vi "publisher.vi"() -> ()   [LabVIEW 2022 SP3]
uses:
  Global 1.vi
panel:
  in  "String":string
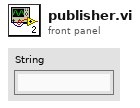
[diagram p1: front panel]
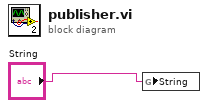
[diagram p0: block diagram]
diagram:
  n1 = global write "Global 1.vi" "String"("String") -> ()
